vi "IMAQ FPGA FIFO to Pixel Bus.vi"   [LabVIEW 2020, in "NI_VDM_FPGA_Basics.lvlib"]
doc: "Reads image pixels out of the specified FIFO and returns a Pixel Bus cluster of the requested type. The Pixel Bus contains the pixel data from the FIFO along with some additional flags that indicate when the pixel data is valid, an end of a line has been reached, or an end of the image has been reached. The Pixel Bus is used to pass image data to all of the other VIs in the NI Vision Development Module for FPGA library. Only one of the DV, EOL, and EOI flags in the Pixel Bus cluster will assert on a given clock cycle. When the last pixel of an image is reached, the Pixel Bus will contain the pixel data and the DV flag will be TRUE and the EOL and EOI flags will be FALSE. The next clock cycle, the EOL flag will be TRUE and the DV and EOI flags will be FALSE. The following clock cycle, the EOI flag will be TRUE and the DV and EOL flags will be FALSE."
uses:
  <vilib>/visionFPGA/NI_VDM_FPGA_Basics.lvlib
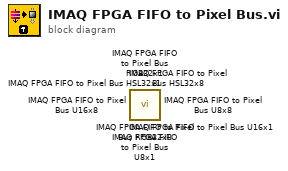
[diagram p0: block diagram]
diagram:
  n1 = call <vilib>:"IMAQ FPGA FIFO to Pixel Bus RGB32x8.vi"() -> ()  [unwired: 9 in, 3 out]
  n2 = call <vilib>:"IMAQ FPGA FIFO to Pixel Bus HSL32x8.vi"() -> ()  [unwired: 9 in, 3 out]
  n3 = call <vilib>:"IMAQ FPGA FIFO to Pixel Bus U16x8.vi"() -> ()  [unwired: 9 in, 3 out]
  n4 = call <vilib>:"IMAQ FPGA FIFO to Pixel Bus U8x8.vi"() -> ()  [unwired: 9 in, 3 out]
  n5 = call <vilib>:"IMAQ FPGA FIFO to Pixel Bus HSL32x1.vi"() -> ()  [unwired: 9 in, 3 out]
  n6 = call <vilib>:"IMAQ FPGA FIFO to Pixel Bus RGB32x1.vi"() -> ()  [unwired: 9 in, 3 out]
  n7 = call <vilib>:"IMAQ FPGA FIFO to Pixel Bus U16x1.vi"() -> ()  [unwired: 9 in, 3 out]
  n8 = call <vilib>:"IMAQ FPGA FIFO to Pixel Bus U8x1.vi"() -> ()  [unwired: 9 in, 3 out]
